vi "Angular Speed Calculation.vi"(7 "reset? (True)":bool=TRUE, 8 "error in (no error)":errorcluster, 9 "avg on n pulses (1:no average)":i32=1, 10 "pulse/revolution (1)":dbl=1.0 format="%.2f", 11 "pulse positions [s]":dbl[](array[numeric]) format="%.2f") -> (0 "error out":errorcluster, 3 "speed profile":T1 {"speed [RPM]" format="%.2f"; "time [s]" format="%.2f"})   [LabVIEW 2017, in "SoundVib_TachProcess.lvlib"]
doc: "Computes the angular speed at each pulse edge contained in <B>pulse positions [s]</B>."
uses:
  <vilib>/addons/Sound and Vibration/Order Analysis/Tach Process/SoundVib_TachProcess.lvlib
  <vilib>/addons/Sound and Vibration/Order Analysis/Tach Process/SubVIs/speed profile.ctl
panel:
  # "Angular Speed (at edges)"
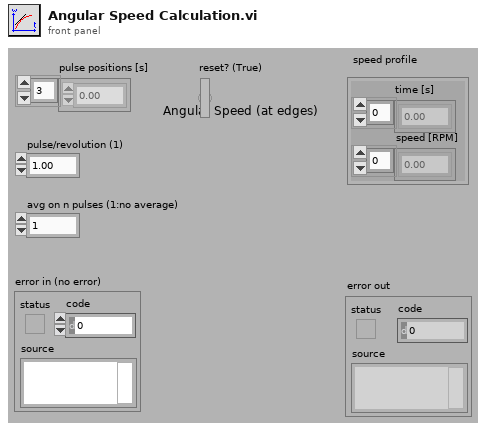
[diagram p1: front panel]
types:
  T1 = typedef "SoundVib_TachProcess.lvlib/speed profile.ctl" = cluster{"time [s]":dbl[], "speed [RPM]":dbl[]}
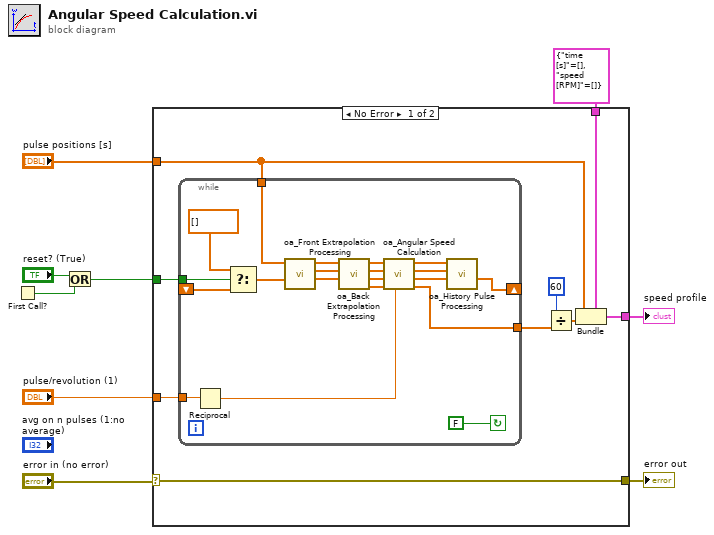
[diagram p0: block diagram]
diagram:
  n1 = First Call?() -> (First Call?: T/F=w3:bool)
  n2 = Or(x="reset? (True)", y=w3) -> (x .or. y?=w1:bool)
  n3 = case shown="No Error" "error in (no error)" {
    selector: "error in (no error)" -> [w10 w39]
    tunnel: "pulse positions [s]" -> [w11 _]
    tunnel: [w17 w40] -> w8
    tunnel: "pulse/revolution (1)" -> [w14 _]
    tunnel: [w10 w39] -> w6
    tunnel: T1 {"time [s]"=[], "speed [RPM]"=[]} ("speed profile") -> [w15 w40]
    tunnel: w1 -> [w12 _]
    frame No Error {
      n4 = while {
        tunnel: [w19] -> w13
        shift-right: [w33] -> _
        shift-left: _ -> [w36]
        tunnel: w14 -> [w37]
        tunnel: w12 -> [w34]
        tunnel: w11 -> [w32]
        stop <- FALSE continue-if-true
        n5 = Reciprocal(x=w37) -> (1/x=w23:dbl)
        n6 = Select(t=dbl[] [] ("empty array"), s=w34, f=w36) -> (s? t:f=w31:dbl[])
        n7 = call <vilib>:"oa_Front Extrapolation Processing.vi"("pulse history in [s]"=w31, "pulse positions in [s]"=w32) -> ("pulse history out [s]"=w29:dbl[], "pulse new history out [s]"=w21:dbl[], "pulse positions out [s]"=w30:dbl[])  [unwired: 7 in]
        n8 = call <vilib>:"oa_Back Extrapolation Processing.vi"("pulse history in [s]"=w29, "pulse new history in [s]"=w21, "pulse positions in [s]"=w30) -> ("pulse future [s]"=w26:dbl[], "pulse history out [s]"=w27:dbl[], "pulse new history out [s]"=w22:dbl[], "pulse positions out [s]"=w28:dbl[])  [unwired: 5 in]
        n9 = call <vilib>:"oa_Angular Speed Calculation.vi"("deltaX"=w23, "pulse future [s]"=w26, "pulse history in  [s]"=w27, "pulse new history in  [s]"=w22, "pulse positions in [s]"=w28) -> ("dY/dX[n]"=w19:dbl[], "pulse history out  [s]"=w24:dbl[], "pulse new history out  [s]"=w20:dbl[], "pulse positions out [s]"=w25:dbl[])  [unwired: 3 in]
        n10 = call <vilib>:"oa_History Pulse Processing.vi"("pulse history in [s]"=w24, "pulse new history in  [s]"=w20, "pulse positions [s]"=w25) -> ("pulse history out [s]"=w33:dbl[])  [unwired: 8 in]
      }
      n11 = Divide(x=60, y=w13) -> (x/y=w16:dbl[])
      n12 = Bundle(cluster=w15, "time [s]"=w11, "speed [RPM]"=w16) -> (w17:T1)
    }
    frame Error {
    }
  }
  "speed profile" <- w8
  "error out" <- w6
